vi "PH_ImageStatistician.Data Collector.vi"(0 "i ref in":refnum<vi>, 2 "Img Op Dataset":T1, 5 "error in (no error)":errorcluster) -> (14 "i ref out":refnum<vi>, 19 "error out":errorcluster)   [LabVIEW 2014, in "PH_ImageStatistician.lvlib"]
doc: "This VI reads the data of the connected image operator."
uses:
  PH_ImageStatistician.lvlib
  PH_ImageStatistician.Statistician Data.ctl
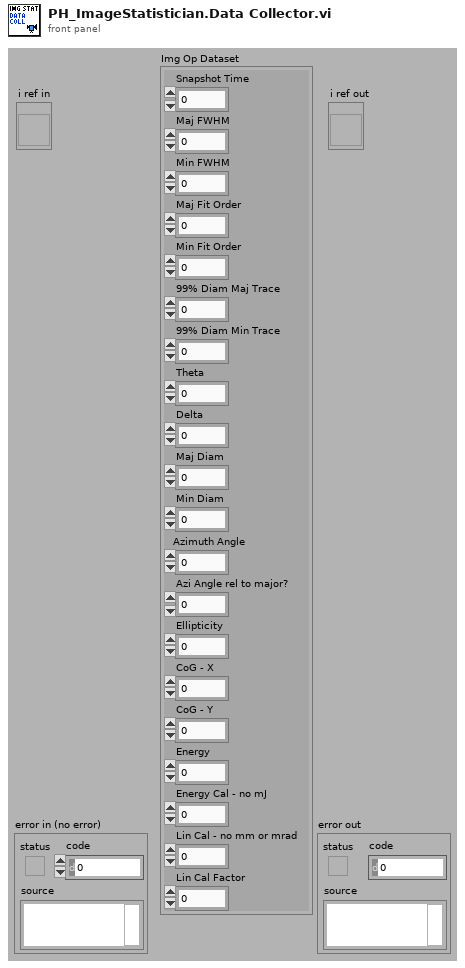
[diagram p1: front panel]
types:
  T1 = typedef "PH_ImageStatistician.lvlib/PH_ImageStatistician.Statistician Data.ctl" = cluster{"Snapshot Time":dbl, "Maj FWHM":dbl, "Min FWHM":dbl, "Maj Fit Order":dbl, "Min Fit Order":dbl, "99% Diam Maj Trace":dbl, "99% Diam Min Trace":dbl, "Theta":dbl, "Delta":dbl, "Maj Diam":dbl, "Min Diam":dbl, "Azimuth Angle":dbl, "Azi Angle rel to major?":dbl, "Ellipticity":dbl, "CoG - X":dbl, "CoG - Y":dbl, "Energy":dbl, "Energy Cal - no mJ":dbl, "Lin Cal - no mm or mrad":dbl, "Lin Cal Factor":dbl}
  T2 = typedef "PH_ImageStatistician.lvlib/PH_ImageStatistician.i attribute.ctl" = cluster{"GUI Refs ":cluster{"Status":refnum<vi>, "Result Graph":refnum<vi>, "Mean Data 1":refnum<vi>, "Std Dev Data 1":refnum<vi>, "Mean Data 2":refnum<vi>, "Std Dev Data 2":refnum<vi>, "Mean Data 3":refnum<vi>, "Std Dev Data 3":refnum<vi>, "Dummy Mean":refnum<vi>, "Dummy Std Dev":refnum<vi>, "Export Data":refnum<vi>, "Data 1":refnum<vi>, "Data 2":refnum<vi>, "Data 3":refnum<vi>, "Stat or Trend":refnum<vi>, "Delete":refnum<vi>, "Operator":refnum<vi>, "Start":refnum<vi>}, "Operator":string, "Data":T1[], "Stat or Trend":bool, "Data 1":T3, "Data 2":T3, "Data 3":T3, "Start":bool, "Datasets strored":i32, "Dataarray Size":i32}
  T3 = typedef "PH_ImageStatistician.lvlib/PH_ImageStatistician.select Data.ctl" = u16
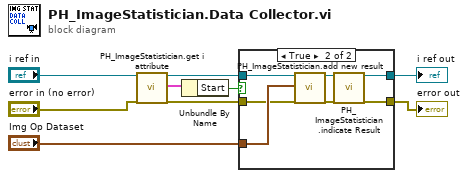
[diagram p0: block diagram]
diagram:
  n1 = call "PH_ImageStatistician.get i attribute.vi"("i ref in"="i ref in", "error in (no error)"="error in (no error)") -> ("i ref out"=w3:refnum<vi>, "i attribute"=w2:T2, "error out"=w5:errorcluster)  [unwired: 15 in]
  n2 = Unbundle By Name(w2) -> ("Start"=w1:bool)
  n3 = case shown="True" w1 {
    tunnel: [w11 w18] -> w9
    tunnel: [w10 w17] -> w8
    tunnel: "Img Op Dataset" -> [_ w16]
    tunnel: w5 -> [w10 w13]
    tunnel: w3 -> [w11 w12]
    frame False {
    }
    frame True {
      n4 = call "PH_ImageStatistician.add new result.vi"("i ref in"=w12, "New Img Op Dataset"=w16, "error in (no error)"=w13) -> ("i ref out"=w14:refnum<vi>, "error out"=w15:errorcluster)  [unwired: 15 in]
      n5 = call "PH_ImageStatistician.indicate Result.vi"("i ref in"=w14, "error in (no error)"=w15) -> ("i ref out"=w18:refnum<vi>, "error out"=w17:errorcluster)  [unwired: 16 in]
    }
  }
  "i ref out" <- w9
  "error out" <- w8
